vi "MenuSelection(User).vi"(6 "User events":T8, 8 "error in":errorcluster {"code" min=0 max=0}, 10 "ItemTag":string, 11 "Data in":T1={"Class"={"Ants"=refnum, "Layer"=refnum, "Templates"=refnum, "Icon"=refnum, "Glyph"=refnum, "Settings"=refnum, "Tools"=refnum}, "Ref"={"Add Layer"=refnum, "Remove Layer"=refnum, "Line Text"=[], "Body Text Spec"=refnum, "DNL_Font"=refnum, "glyph path str"=refnum, "templates path str"=refnum, "Arrow Up"=refnum, "Arrow Down"=refnum, "IE VI Ref"=refnum, "Glyphs tree"=refnum, "Templates tree"=refnum, "Layer Icon Text"=refnum, "Layer Template"=refnum, "Clipboard"=refnum, "BW icon in"=refnum, "Color icon in"=refnum, "Layer Clust"=refnum, "Body Text"=refnum, "DNL_Framework Templates"=refnum, "Search Templates"=refnum, "TextMarker"=refnum, "Tab Control"=refnum, "Search Glyphs"=refnum, "Line Color"=refnum, "DNL_Glyphs []"=refnum, "Fill Color"=refnum, "Tools"=refnum, "Glyphs tree"=refnum, "Icon"=refnum, "Preview"=refnum, "Ants"=refnum, "Terminals"=refnum, "menu reference"=refnum, "LayerNames"=[], "GlyphLoadAnimation"=refnum, "TemplateLoadAnimation"=refnum, "refreshGlyphs"=refnum, "refreshTemplates"=refnum}, "Support"={"AntsRect"={"left"=0, "top"=0, "right"=0, "bottom"=0}, "Mouse Move Coords"={"Horizontal"=0, "Vertical"=0}, "Mouse Down Coords"={"Horizontal"=0, "Vertical"=0}, "Temp Coord"={"Horizontal"=0, "Vertical"=0}, "Action"=enum."Default", "Edge Color"=4914962, "Fill Color"=16860, "Mouse Down?"=FALSE, "Draft Mode?"=FALSE, "Temp Icon"=bytes[3102], "CTRL Pressed"=FALSE, "Move Selection?"=FALSE, "AntsRect Orig"={"left"=0, "top"=0, "right"=0, "bottom"=0}, "Text"="", "TM Set?"=FALSE, "Mouse inside icon?"=FALSE, "Tool (old value)"=0, "Pencil Move Color"=0, "Swap Colors?"=FALSE, "Shift pressed?"=FALSE}}) -> (0 "error out":errorcluster {"code" min=0 max=0}, 3 "Data out":T1={"Class"={"Ants"=refnum, "Layer"=refnum, "Templates"=refnum, "Icon"=refnum, "Glyph"=refnum, "Settings"=refnum, "Tools"=refnum}, "Ref"={"Add Layer"=refnum, "Remove Layer"=refnum, "Line Text"=[], "Body Text Spec"=refnum, "DNL_Font"=refnum, "glyph path str"=refnum, "templates path str"=refnum, "Arrow Up"=refnum, "Arrow Down"=refnum, "IE VI Ref"=refnum, "Glyphs tree"=refnum, "Templates tree"=refnum, "Layer Icon Text"=refnum, "Layer Template"=refnum, "Clipboard"=refnum, "BW icon in"=refnum, "Color icon in"=refnum, "Layer Clust"=refnum, "Body Text"=refnum, "DNL_Framework Templates"=refnum, "Search Templates"=refnum, "TextMarker"=refnum, "Tab Control"=refnum, "Search Glyphs"=refnum, "Line Color"=refnum, "DNL_Glyphs []"=refnum, "Fill Color"=refnum, "Tools"=refnum, "Glyphs tree"=refnum, "Icon"=refnum, "Preview"=refnum, "Ants"=refnum, "Terminals"=refnum, "menu reference"=refnum, "LayerNames"=[], "GlyphLoadAnimation"=refnum, "TemplateLoadAnimation"=refnum, "refreshGlyphs"=refnum, "refreshTemplates"=refnum}, "Support"={"AntsRect"={"left"=0, "top"=0, "right"=0, "bottom"=0}, "Mouse Move Coords"={"Horizontal"=0, "Vertical"=0}, "Mouse Down Coords"={"Horizontal"=0, "Vertical"=0}, "Temp Coord"={"Horizontal"=0, "Vertical"=0}, "Action"=enum."Default", "Edge Color"=4914962, "Fill Color"=16860, "Mouse Down?"=FALSE, "Draft Mode?"=FALSE, "Temp Icon"=bytes[3102], "CTRL Pressed"=FALSE, "Move Selection?"=FALSE, "AntsRect Orig"={"left"=0, "top"=0, "right"=0, "bottom"=0}, "Text"="", "TM Set?"=FALSE, "Mouse inside icon?"=FALSE, "Tool (old value)"=0, "Pencil Move Color"=0, "Swap Colors?"=FALSE, "Shift pressed?"=FALSE}})   [LabVIEW 2021]
uses:
  Controls/IE Data.ctl
  Class/Ants/Ants.lvclass
  Class/FakedArray/FakedArray.lvclass
  vi.lib/LabVIEW Icon API/lv_icon/Classes/Icon/Icon.lvclass
  Class/Icon Library/Glyph.lvclass
  Class/Settings/Settings.lvclass
  Class/Tools/Tools Paint.lvclass
  Controls/IE Classes.ctl
  Controls/References Cluster.ctl
  Controls/SupportClass.ctl
  <vilib>/Utility/miscctls.llb/LVPoint32TypeDef.ctl
  Controls/SupportClass_Action.ctl
  vi.lib/LabVIEW Icon API/lv_icon/Controls/IEColor.ctl
  vi.lib/LabVIEW Icon API/lv_icon/Controls/Pathes.ctl
  vi.lib/LabVIEW Icon API/lv_icon/Controls/Graphic.ctl
  vi.lib/LabVIEW Icon API/lv_icon/Classes/Icon Framework/Icon Framework.lvclass
  vi.lib/LabVIEW Icon API/lv_icon/Classes/Layer/Layer.lvclass
  vi.lib/LabVIEW Icon API/lv_icon/Controls/Layer.ctl
  Controls/Undo Redo Action.ctl
  Controls/Tools.ctl
  vi.lib/LabVIEW Icon API/lv_icon/lv_icon.lvlib
panel:
  in  "Layer name":string="Clipboard"
  in  "glyph":string="Glyph name"
  in  "template":string="Template name"
  in  "Prompt":string="Save Glyph"
  in  "prompt":string="Save Icon Template"
  in  "LayerName":string="Merged Layers"
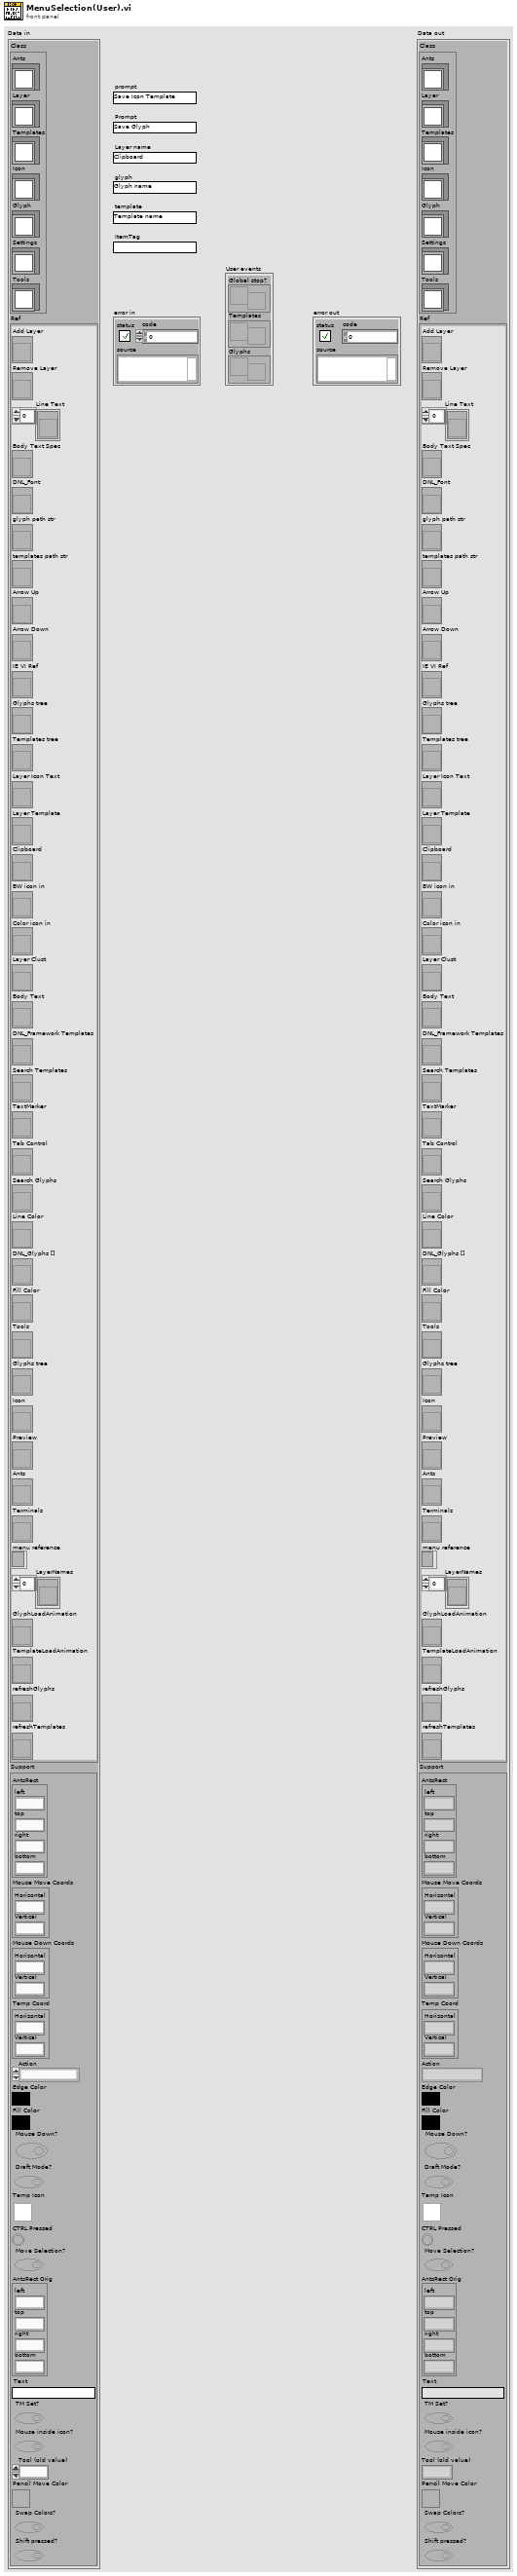
[diagram p1: front panel]
types:
  T1 = typedef "IE Data.ctl" = cluster{"Class":T2, "Ref":T3, "Support":T4}
  T2 = typedef "IE Classes.ctl" = cluster{"Ants":refnum<class "Ants.lvclass">, "Layer":refnum<class "FakedArray.lvclass">, "Templates":refnum<class "FakedArray.lvclass">, "Icon":refnum<class "Icon.lvclass">, "Glyph":refnum<class "Glyph.lvclass">, "Settings":refnum<class "Settings.lvclass">, "Tools":refnum<class "Tools Paint.lvclass">}
  T3 = typedef "References Cluster.ctl" = cluster{"Add Layer":refnum<vi>, "Remove Layer":refnum<vi>, "Line Text":refnum<vi>[], "Body Text Spec":refnum<vi>, "DNL_Font":refnum<vi>, "glyph path str":refnum<vi>, "templates path str":refnum<vi>, "Arrow Up":refnum<vi>, "Arrow Down":refnum<vi>, "IE VI Ref":refnum<vi>, "Glyphs tree":refnum<vi>, "Templates tree":refnum<vi>, "Layer Icon Text":refnum<vi>, "Layer Template":refnum<vi>, "Clipboard":refnum<vi>, "BW icon in":refnum<vi>, "Color icon in":refnum<vi>, "Layer Clust":refnum<vi>, "Body Text":refnum<vi>, "DNL_Framework Templates":refnum<vi>, "Search Templates":refnum<vi>, "TextMarker":refnum<vi>, "Tab Control":refnum<vi>, "Search Glyphs":refnum<vi>, "Line Color":refnum<vi>, "DNL_Glyphs []":refnum<vi>, "Fill Color":refnum<vi>, "Tools":refnum<vi>, "Glyphs tree":refnum<vi>, "Icon":refnum<vi>, "Preview":refnum<vi>, "Ants":refnum<vi>, "Terminals":refnum<vi>, "menu reference":refnum<k9>, "LayerNames":refnum<vi>[], "GlyphLoadAnimation":refnum<vi>, "TemplateLoadAnimation":refnum<vi>, "refreshGlyphs":refnum<vi>, "refreshTemplates":refnum<vi>}
  T4 = typedef "SupportClass.ctl" = cluster{"AntsRect":cluster{"left":i16, "top":i16, "right":i16, "bottom":i16}, "Mouse Move Coords":T5, "Mouse Down Coords":T5, "Temp Coord":T5, "Action":T6, "Edge Color":T7, "Fill Color":T7, "Mouse Down?":bool, "Draft Mode?":bool, "Temp Icon":picture, "CTRL Pressed":bool, "Move Selection?":bool, "AntsRect Orig":cluster{"left":i16, "top":i16, "right":i16, "bottom":i16}, "Text":string, "TM Set?":bool, "Mouse inside icon?":bool, "Tool (old value)":u32, "Pencil Move Color":u32, "Swap Colors?":bool, "Shift pressed?":bool}
  T5 = typedef "LVPoint32TypeDef.ctl" = cluster{"Horizontal":i32, "Vertical":i32}
  T6 = typedef "SupportClass_Action.ctl" = enum16{"Default", "Move Selection", "Glyph Library", "Tool"}
  T7 = typedef "IEColor.ctl" = u32
  T8 = cluster{"Global stop?":refnum<user-event>, "Templates":refnum<user-event>, "Glyphs":refnum<user-event>}
  T9 = typedef "Pathes.ctl" = enum16{"Root Path", "Icon Templates", "Icon Templates VI", "Icon Templates Lib", "Glyphs"}
  T10 = typedef "Graphic.ctl" = cluster{"Rectangle":cluster{"left":i16, "top":i16, "right":i16, "bottom":i16}, "Path":path, "Image":picture, "Filter":string, "FileName":string}
  T11 = typedef "Layer.ctl" = cluster{"LayerIcon":picture, "LayerName":string, "Opacity":u8, "Visibility?":bool}
  T12 = typedef "Undo Redo Action.ctl" = enum16{"Init", "Add", "Redo", "Undo", "Undo Preview"}
  T13 = enum32{"Pencil", "Line", "Dropper", "Fill", "Rectangle", "Filled Rectangle", "Ellipse", "Filled Ellipse", "Eraser", "Text", "Select", "Move"}
  T14 = typedef "Tools.ctl" = enum32{"Pencil", "Line", "Dropper", "Fill", "Rectangle", "Filled Rectangle", "Ellipse", "Filled Ellipse", "Eraser", "Text", "Select", "Move"}
  T15 = typedef "imagedata.ctl" = cluster{"image type":i32, "image depth":i32, "image":u8[], "mask":u8[], "colors":u32[], "Rectangle":cluster{"left":i16, "top":i16, "right":i16, "bottom":i16}}
  T16 = typedef "Font.ctl" = string
  T17 = typedef "Alignment.ctl" = u16
  T18 = typedef "Font Size.ctl" = u8
  T19 = cluster{"Line 1 text":string, "Line 2 text":string, "Line 3 text":string, "Line 4 text":string, "Line 1 color":u32, "Line 2 color":u32, "Line 3 color":u32, "Line 4 color":u32, "Body Text Spec":cluster{"DNL_Font":T16, "Alignment":T17, "Size":T18}, "Center text vertically":bool, "Capitalize Text":bool}
  T20 = cluster{"left":i16, "top":i16, "right":i16, "bottom":i16}
  T21 = cluster{"Horizontal":i32, "Vertical":i32, "Vertical 2":i32, "Vertical 3":i32}
  T22 = cluster{"Left":i32, "Top":i32, "Right":i32, "Bottom":i32}
  T23 = typedef "Icon Editor Invoker Type.ctl" = enum32{"Unknown Icon Source", "VI Icon", "Library Icon (any library type)", "Palette icon", "Icon from App Method"}
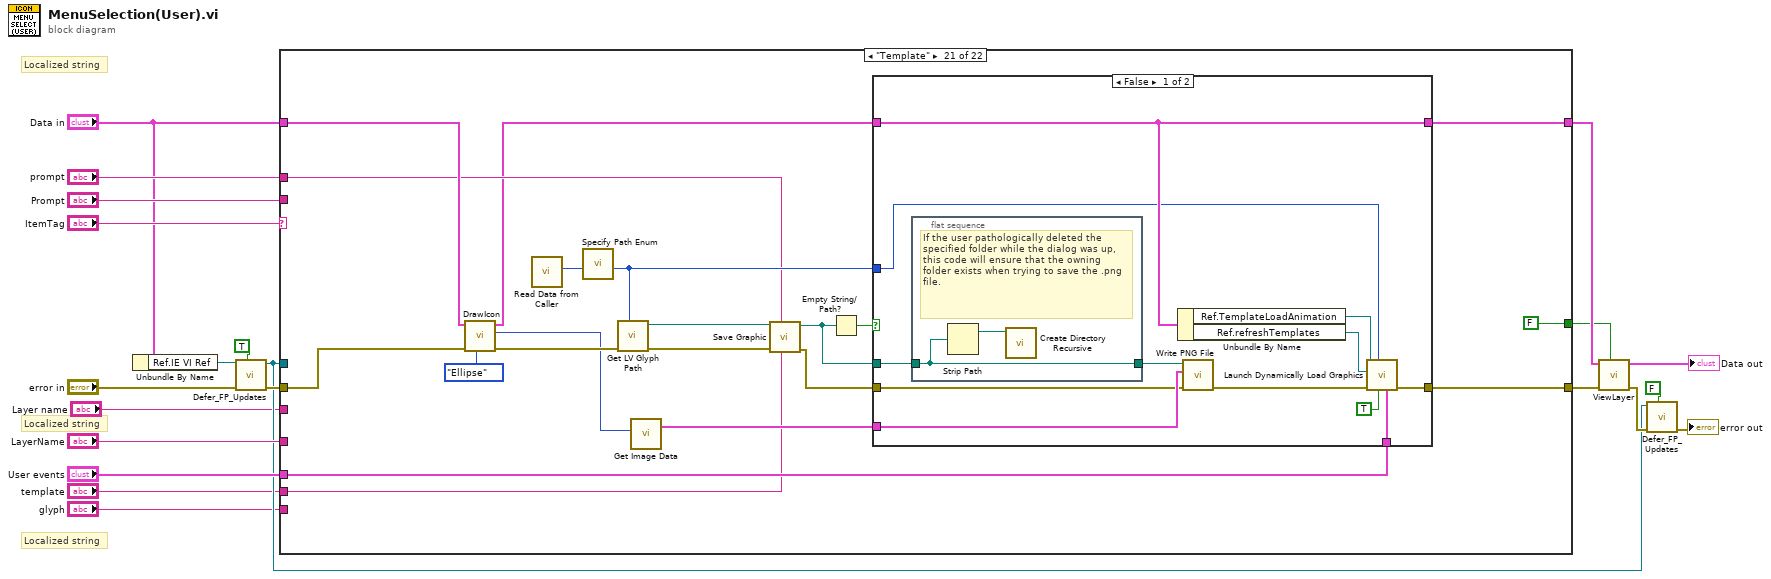
[diagram p0: block diagram]
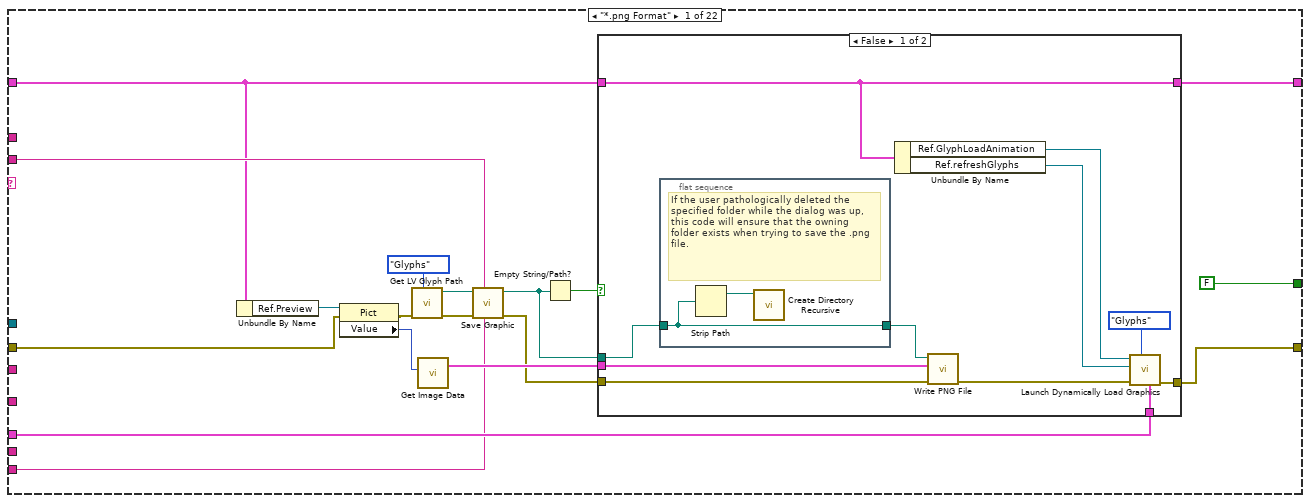
[diagram p2: hidden frame]
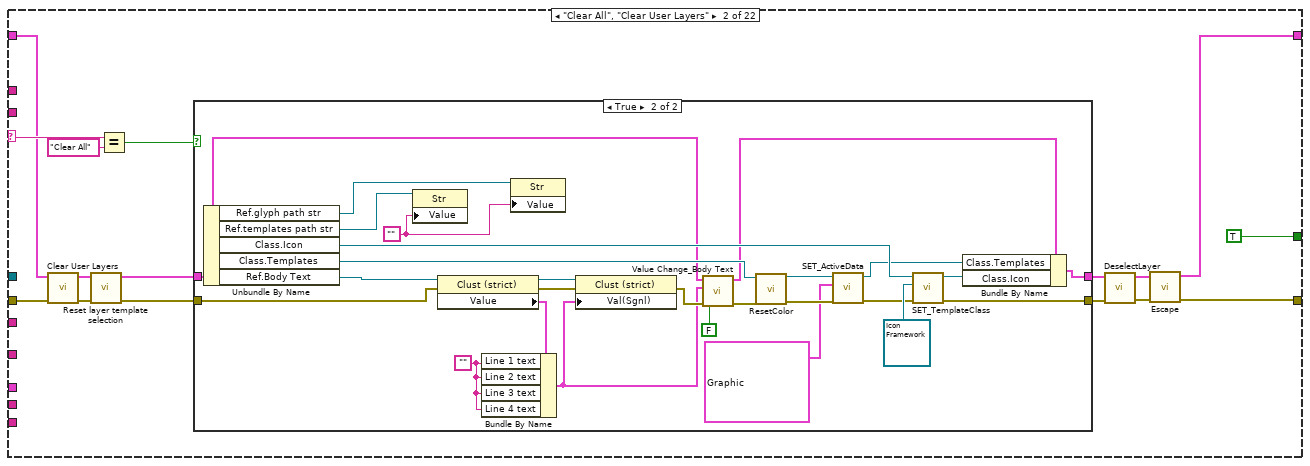
[diagram p4: hidden frame]
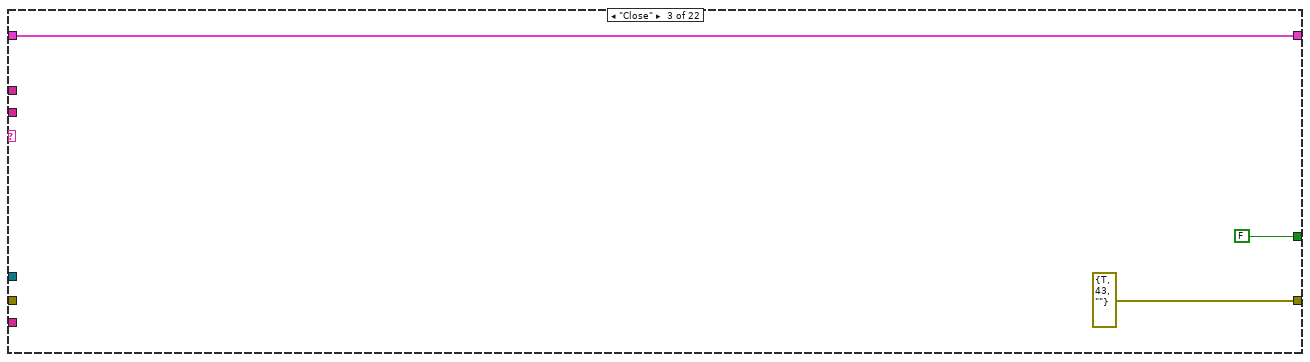
[diagram p6: hidden frame]
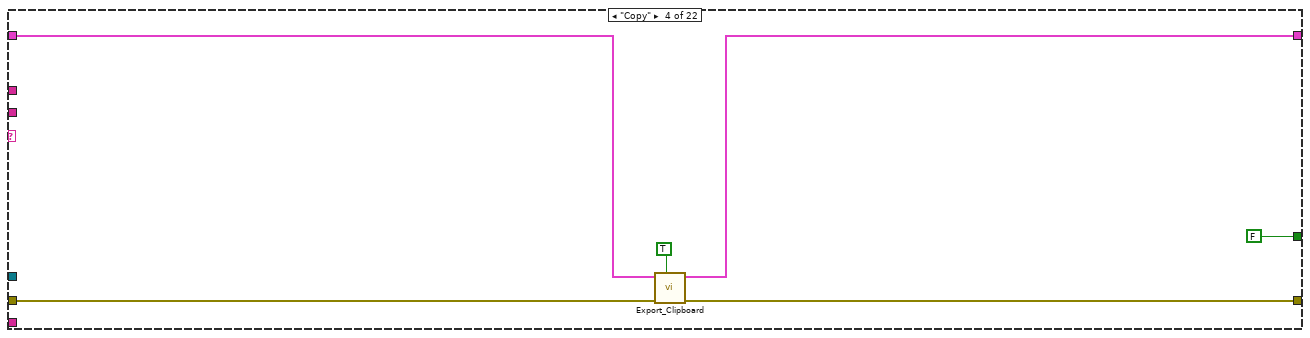
[diagram p7: hidden frame]
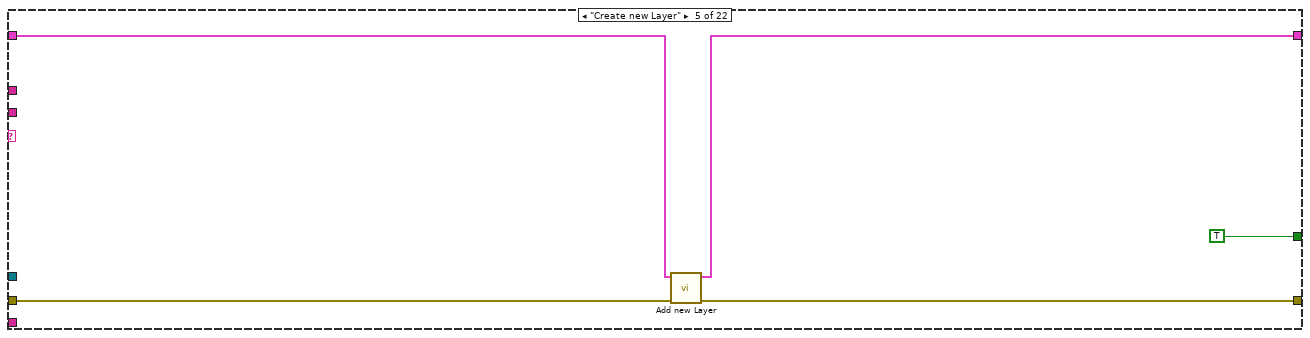
[diagram p8: hidden frame]
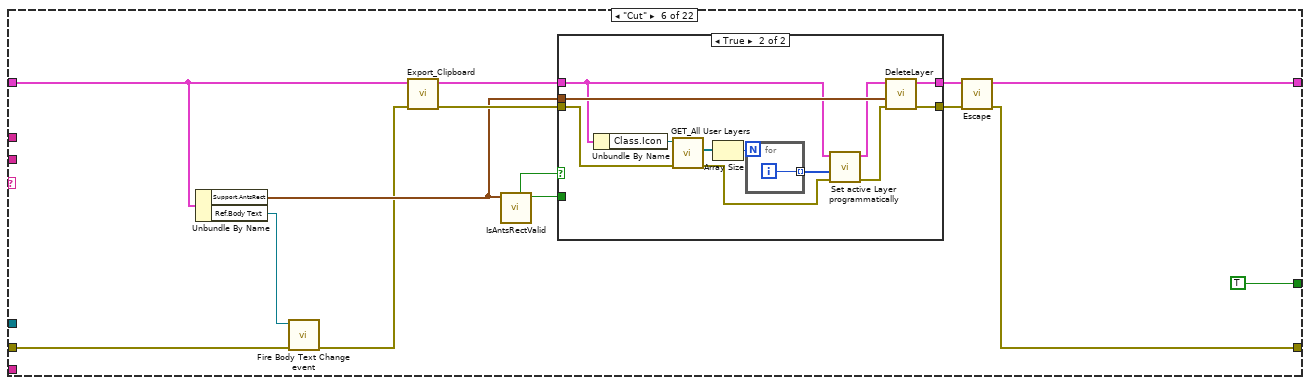
[diagram p9: hidden frame]
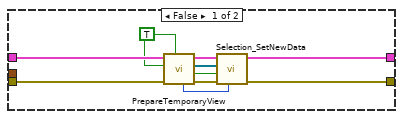
[diagram p10: hidden frame]
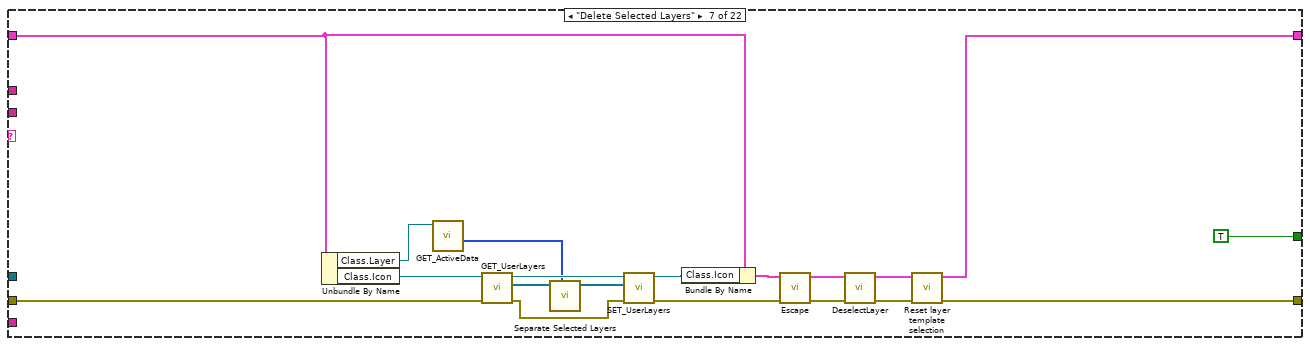
[diagram p11: hidden frame]
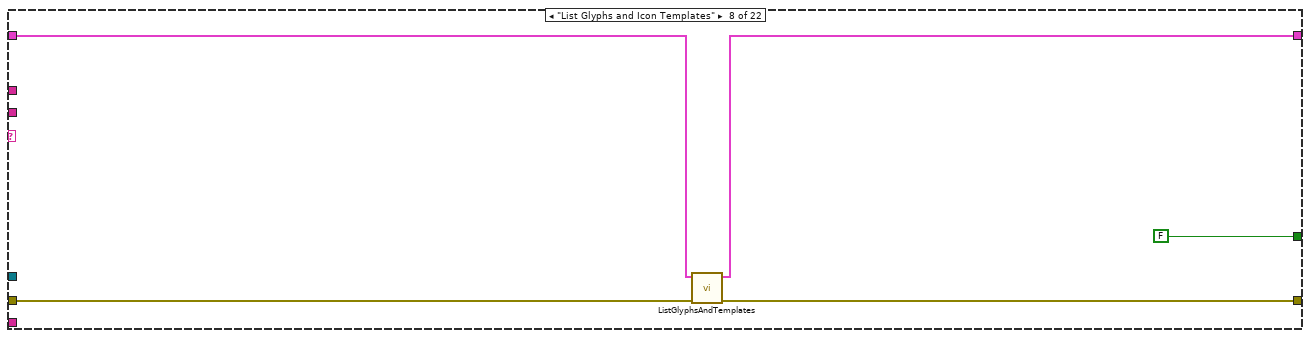
[diagram p12: hidden frame]
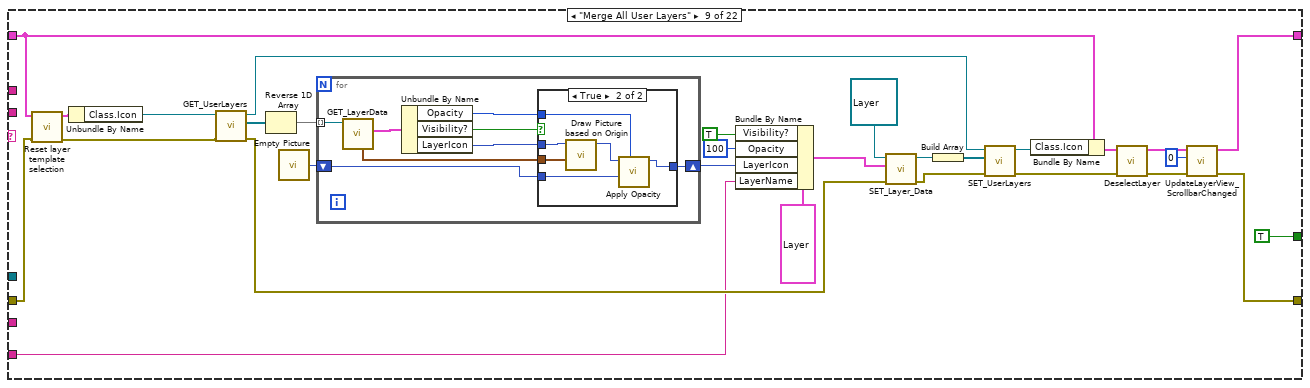
[diagram p13: hidden frame]
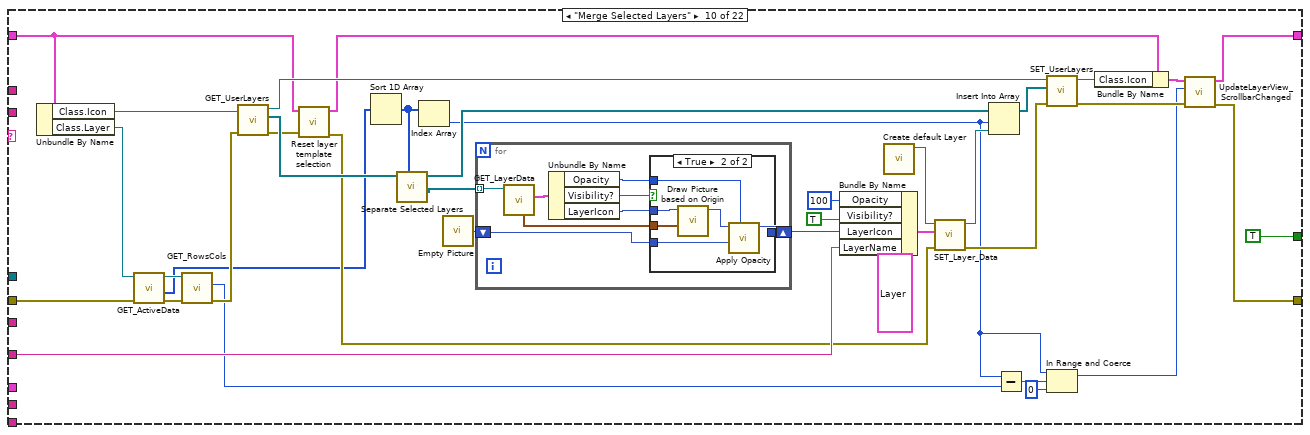
[diagram p15: hidden frame]
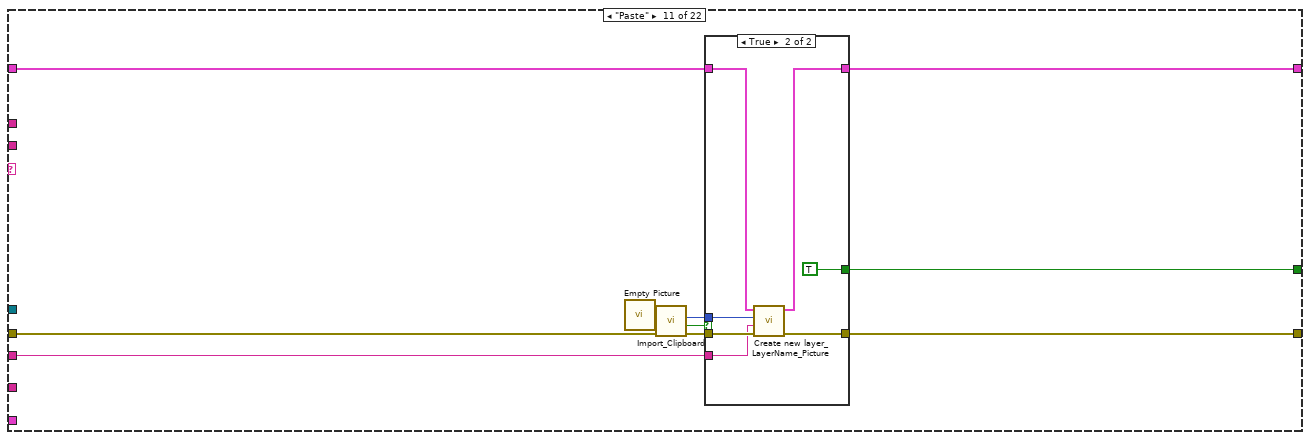
[diagram p17: hidden frame]
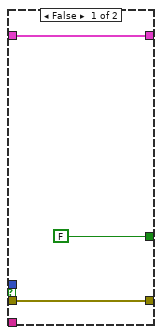
[diagram p18: hidden frame]
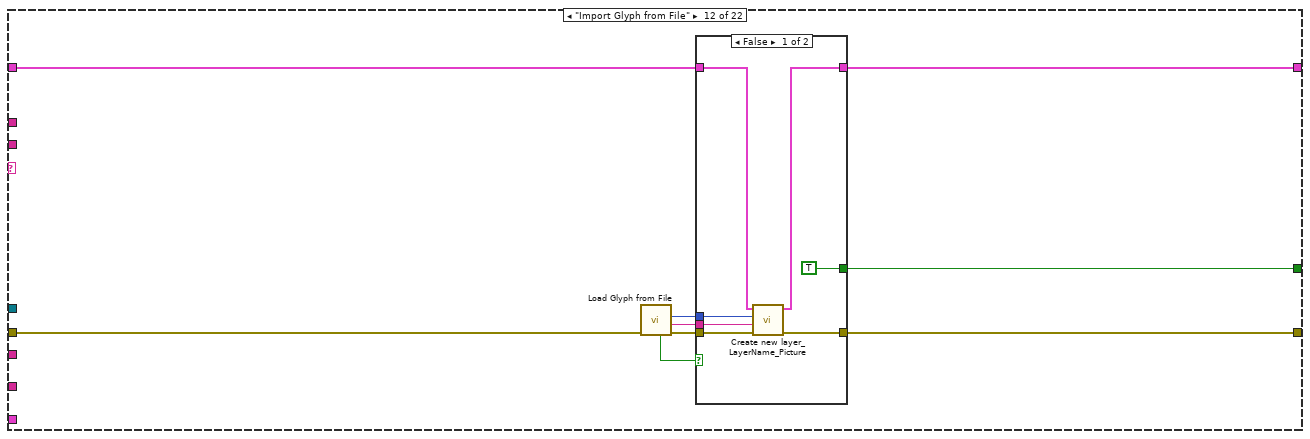
[diagram p19: hidden frame]
diagram:
  # "Localized string"
  # "Localized string"
  # "Localized string"
  n1 = Unbundle By Name("Data in") -> ("Ref.IE VI Ref"=w8:refnum<vi>)
  n2 = call "Defer_FP_Updates.vi"("Defer Panel Updates"=TRUE, "error in (no error)"="error in", "lv_icon.vi in"=w8) -> ("error out"=w11:errorcluster, "lv icon.vi out"=w4:refnum<vi>)  [unwired: 7 out]
  n3 = case shown="\"Template\"" "ItemTag" {
    selector: "ItemTag" -> [_ w70 _ _ _ _ _ _ _ _ _ _ _ w340 _ w388 _ _ _ _ _ _]
    tunnel: w11 -> [w26 w59 _ w107 w108 w115 w160 w173 w188 w219 w275 w296 w321 w325 w373 w378 w397 w400 w415 w438 w461 w493]
    tunnel: [w27 w62 errorcluster {"status"=TRUE, "code"=43, "source"=""} ("Icon 43") w106 w109 w125 w150 w172 w175 w231 w278 w298 w312 w331 w354 w380 w390 w402 w416 w445 w460 w493] -> w16
    tunnel: "LayerName" -> [_ _ _ _ _ _ _ _ w190 w244 _ _ _ _ _ _ _ _ _ _ _ _]
    tunnel: "prompt" -> [_ _ _ _ _ _ _ _ _ _ _ _ _ _ _ _ _ _ _ _ w463 _]
    tunnel: "Prompt" -> [w28 _ _ _ _ _ _ _ _ _ _ _ _ _ _ _ _ _ _ _ _ _]
    tunnel: [FALSE TRUE FALSE FALSE TRUE TRUE TRUE FALSE TRUE TRUE w280 w291 TRUE FALSE FALSE FALSE FALSE FALSE FALSE FALSE FALSE FALSE] -> w13
    tunnel: "User events" -> [w33 _ _ _ _ _ _ _ _ _ _ _ _ _ _ _ _ _ _ w443 w469 _]
    tunnel: [w22 w63 w99 w104 w111 w124 w153 w169 w176 w233 w277 w297 w309 w323 w355 w379 w389 w403 w414 w429 w456 w491] -> w14
    tunnel: "Data in" -> [w23 w60 w99 w103 w110 w119 w155 w170 w184 w236 w279 w299 w311 w327 w369 w381 w396 w405 w419 w430 w466 w491]
    tunnel: w4 -> [_ _ _ _ _ _ _ _ _ _ _ _ _ _ _ _ _ w399 _ _ _ _]
    tunnel: "template" -> [_ _ _ _ _ _ _ _ _ _ _ _ _ _ _ _ _ _ _ _ w458 _]
    tunnel: "glyph" -> [w24 _ _ _ _ _ _ _ _ _ _ _ _ _ _ _ _ _ _ _ _ _]
    tunnel: "Layer name" -> [_ _ _ _ _ _ _ _ _ _ w271 _ _ _ _ _ _ _ _ _ _ _]
    frame "*.png Format" {
      n4 = Unbundle By Name(w23) -> ("Ref.Preview"=w39:refnum<vi>)
      n5 = property class="Pict"(reference=w39, error in=w26) -> (error out=w35:errorcluster, "Value"=w37:picture)  [unwired: 1 out]
      n6 = call "Get LV Glyph Path.vi"("Path"=Pathes."Glyphs", "error in (no error)"=w35) -> ("error out"=w32:errorcluster, "Requested Path"=w29:path)  [unwired: 1 in, 7 out]
      n7 = call "Get Image Data.vi"("Pic In"=w37) -> ("image data out"=w38:T15)  [unwired: 3 in, 7 out]
      n8 = call "Save Graphic.vi"("Loc string caption"=w24, "FP Title"=w28, "error in (no error)"=w32, "Start path in"=w29) -> ("error out"=w31:errorcluster, "Output"=w30:path)  [unwired: 6 out]
      n9 = Empty String/Path?(string/path=w30) -> (empty?=w25:bool)
      n10 = case shown="False" w25 {
        tunnel: w38 -> [w50 _]
        tunnel: w33 -> [w47 _]
        tunnel: w31 -> [w46 w54]
        tunnel: w30 -> [w41 _]
        tunnel: [w45 w54] -> w27
        tunnel: w23 -> [w44 w53]
        tunnel: [w44 w53] -> w22
        frame False {
          n11 = flat-sequence {
            tunnel: w41 -> [w52]
            tunnel: [w52] -> w40
            frame #0 {
              # "If the user pathologically deleted the specified folder while the dialog was up, this code will ensure that the owning folder exists when trying to save the .png file."
              n12 = Strip Path(path=w52) -> (stripped path=w51:path)  [unwired: 1 out]
              n13 = call <vilib>:"Create Directory Recursive.vi"("directory"=w51) -> ()  [unwired: 4 in, 3 out]
            }
          }
          n14 = Unbundle By Name(w44) -> ("Ref.GlyphLoadAnimation"=w42:refnum<vi>, "Ref.refreshGlyphs"=w43:refnum<vi>)
          n15 = call <vilib>:"Write PNG File.vi"("error in (no error)"=w46, "image data"=w50, "path to PNG file"=w40) -> ("error out"=w49:errorcluster)  [unwired: 1 in, 7 out]
          n16 = call "Launch Dynamically Load Graphics.vi"("User events"=w47, "Path"=Pathes."Glyphs", "error in (no error)"=w49, "button ref"=w43, "animatedDecoration ref"=w42) -> ("error out"=w45:errorcluster)  [unwired: 1 in, 5 out]
        }
        frame True {
        }
      }
    }
    frame "Clear All", "Clear User Layers" {
      n17 = call "Clear User Layers.vi"("error in"=w59, "Data in"=w60) -> ("error out"=w58:errorcluster, "Data out"=w57:T1)  [unwired: 8 out]
      n18 = call "Reset layer template selection.vi"("error in (no error)"=w58, "Data in"=w57) -> ("error out"=w55:errorcluster, "Data out"=w56:T1)  [unwired: 1 in, 7 out]
      n19 = Equal?(x=w70, y="Clear All") -> (x = y?=w69:bool)
      n20 = case shown="True" w69 {
        tunnel: w55 -> [w72 w86]
        tunnel: w56 -> [w71 w77]
        tunnel: [w72 w80] -> w67
        tunnel: [w71 w78] -> w65
        frame False {
        }
        frame True {
          w73 = ""
          w94 = ""
          n21 = Unbundle By Name(w77) -> ("Ref.glyph path str"=w74:refnum<vi>, "Ref.templates path str"=w75:refnum<vi>, "Class.Icon"=w83:refnum<class "Icon.lvclass">, "Class.Templates"=w85:refnum<class "FakedArray.lvclass">, "Ref.Body Text"=w98:refnum<vi>)
          n22 = property class="Str"(reference=w75, "Value"=w73) -> ()  [unwired: 1 in, 2 out]
          n23 = property class="Clust (strict)"(reference=w98, error in=w86) -> (reference out=w97:refnum<vi>, error out=w96:errorcluster, "Value"=w95:T19)
          n24 = Bundle By Name(cluster=w95, "Line 1 text"=w94, "Line 2 text"=w94, "Line 3 text"=w94, "Line 4 text"=w94) -> (w87:T19)
          n25 = property class="Str"(reference=w74, "Value"=w73) -> ()  [unwired: 1 in, 2 out]
          n26 = property class="Clust (strict)"(reference=w97, error in=w96, "Val(Sgnl)"=w87) -> (error out=w89:errorcluster)  [unwired: 1 out]
          n27 = call "Value Change_Body Text.vi"("Add to Undo?"=FALSE, "error in"=w89, "NewVal"=w87, "Data in"=w77) -> ("error out"=w84:errorcluster, "Data out"=w76:T1)  [unwired: 1 in, 5 out]
          n28 = call "ResetColor.vi"("error in (no error)"=w84, "FakedArray in"=w85) -> ("error out"=w92:errorcluster, "FakedArray out"=w93:refnum<class "FakedArray.lvclass">)  [unwired: 8 out]
          n29 = call-dynamic "SET_ActiveData.vi"("error in (no error)"=w92, "Active Data"=T10 {"Rectangle"={"left"=0, "top"=0, "right"=0, "bottom"=0}, "Path"=path "", "Image"=bytes[0], "Filter"="", "FileName"=""} ("Path & Icon"), "FakedArray.lvclass in"=w93) -> ("error out"=w82:errorcluster, "FakedArray.lvclass out"=w79:refnum<class "FakedArray.lvclass">)  [unwired: 7 out]
          n30 = call-dynamic "SET_TemplateClass.vi"("error in (no error)"=w82, "Icon Framework.lvclass"=refnum<class "Icon Framework.lvclass"> refnum ("lv_icon.lvlib:Icon Framework.lvclass"), "Icon.lvclass in"=w83) -> ("error out"=w80:errorcluster, "Icon.lvclass out"=w81:refnum<class "Icon.lvclass">)  [unwired: 7 out]
          n31 = Bundle By Name(cluster=w76, "Class.Templates"=w79, "Class.Icon"=w81) -> (w78:T1)
        }
      }
      n32 = call "DeselectLayer.vi"("error in (no error)"=w67, "Data in"=w65) -> ("error out"=w61:errorcluster, "Data out"=w64:T1)  [unwired: 8 out]
      n33 = call "Escape.vi"("error in"=w61, "Data in"=w64) -> ("error out"=w62:errorcluster, "Data out"=w63:T1)  [unwired: 2 in, 6 out]
    }
    frame "Close" {
    }
    frame "Copy" {
      n34 = call "Export_Clipboard.vi"("Is Copy? (F)"=TRUE, "error in (no error)"=w107, "Data in"=w103) -> ("error out"=w106:errorcluster, "Data out"=w104:T1)  [unwired: 7 out]
    }
    frame "Create new Layer" {
      n35 = call "Add new Layer.vi"("error in"=w108, "Data in"=w110) -> ("error out"=w109:errorcluster, "Data out"=w111:T1)  [unwired: 8 out]
    }
    frame "Cut" {
      n36 = Unbundle By Name(w119) -> ("Support.AntsRect"=w118:T20, "Ref.Body Text"=w116:refnum<vi>)
      n37 = call "Fire Body Text Change event.vi"("error in"=w115, "Ref.Body Text"=w116) -> ("error out"=w114:errorcluster)  [unwired: 2 in, 7 out]
      n38 = call "Export_Clipboard.vi"("error in (no error)"=w114, "Data in"=w119) -> ("error out"=w121:errorcluster, "Data out"=w120:T1)  [unwired: 8 out]
      n39 = call "IsAntsRectValid.vi"("AntsRect"=w118) -> ("Valid?"=w122:bool, "Max. Rect size?"=w123:bool)  [unwired: 9 out]
      n40 = case shown="True" w123 {
        tunnel: w122 -> [_ _]
        tunnel: w120 -> [w136 w140]
        tunnel: [w135 w147] -> w113
        tunnel: [w134 w148] -> w117
        tunnel: w121 -> [w127 w138]
        tunnel: w118 -> [_ w146]
        frame False {
          w133 = TRUE ("Delete Selected Area?")
          n41 = call "PrepareTemporaryView.vi"("Delete Selected Area?"=w133, "error in (no error)"=w127, "Valid Selection?"=w133, "Data in"=w136) -> ("error out"=w130:errorcluster, "Highlighted?"=w131:bool, "All Layers out"=w132:refnum<class "Layer.lvclass">[], "Data out"=w128:T1, "#Active Layer"=w129:i32)  [unwired: 1 in, 2 out]
          n42 = call "Selection_SetNewData.vi"("#Active Layer"=w129, "error in"=w130, "Highlighted?"=w131, "All Layers In"=w132, "Data in"=w128) -> ("error out"=w135:errorcluster, "Data out"=w134:T1)  [unwired: 1 in, 3 out]
        }
        frame True {
          n43 = Unbundle By Name(w140) -> ("Class.Icon"=w145:refnum<class "Icon.lvclass">)
          n44 = call-dynamic "GET_All User Layers.vi"("error in (no error)"=w138, "Icon.lvclass in"=w145) -> ("error out"=w144:errorcluster, "User Layer"=w141:refnum<class "Layer.lvclass">[])  [unwired: 7 in, 1 out]
          n45 = Array Size(array=w141) -> (size(s)=w142:i32)
          n46 = for {
            N: w142 -> [_]
            tunnel: [w149] -> w143 mode=indexing
            i -> [w149]
          }
          n47 = call "Set active Layer programmatically.vi"("error in"=w144, "Active Layer []"=w143, "Data in"=w140) -> ("error out"=w137:errorcluster, "Data out"=w139:T1)  [unwired: 7 in]
          n48 = call "DeleteLayer.vi"("error in"=w137, "AntsRect"=w146, "Data in"=w139) -> ("error out"=w147:errorcluster, "Data out"=w148:T1)  [unwired: 5 out]
        }
      }
      n49 = call "Escape.vi"("error in"=w113, "Data in"=w117) -> ("error out"=w125:errorcluster, "Data out"=w124:T1)  [unwired: 2 in, 6 out]
    }
    frame "Delete Selected Layers" {
      n50 = Unbundle By Name(w155) -> ("Class.Layer"=w152:refnum<class "FakedArray.lvclass">, "Class.Icon"=w163:refnum<class "Icon.lvclass">)
      n51 = call-dynamic "GET_ActiveData.vi"("FakedArray in"=w152) -> ("Active Data []"=w161:i32[])  [unwired: 1 in, 9 out]
      n52 = call-dynamic "GET_UserLayers.vi"("error in (no error)"=w160, "Icon.lvclass in"=w163) -> ("error out"=w164:errorcluster, "All Layers"=w168:refnum<class "Layer.lvclass">[], "Icon.lvclass out"=w167:refnum<class "Icon.lvclass">)  [unwired: 7 out]
      n53 = call "Separate Selected Layers.vi"("Active Indices"=w161, "All Layers"=w168) -> ("Layers out not in Array"=w166:refnum<class "Layer.lvclass">[])  [unwired: 9 out]
      n54 = call-dynamic "SET_UserLayers.vi"("error in (no error)"=w164, "Layers"=w166, "Icon.lvclass in"=w167) -> ("error out"=w151:errorcluster, "Icon.lvclass out"=w162:refnum<class "Icon.lvclass">)  [unwired: 7 in]
      n55 = Bundle By Name(cluster=w155, "Class.Icon"=w162) -> (w154:T1)
      n56 = call "Escape.vi"("error in"=w151, "Data in"=w154) -> ("error out"=w159:errorcluster, "Data out"=w158:T1)  [unwired: 8 out]
      n57 = call "DeselectLayer.vi"("error in (no error)"=w159, "Data in"=w158) -> ("error out"=w156:errorcluster, "Data out"=w157:T1)  [unwired: 8 out]
      n58 = call "Reset layer template selection.vi"("error in (no error)"=w156, "Data in"=w157) -> ("error out"=w150:errorcluster, "Data out"=w153:T1)  [unwired: 1 in, 7 out]
    }
    frame "List Glyphs and Icon Templates" {
      n59 = call "ListGlyphsAndTemplates.vi"("error in"=w173, "Data in"=w170) -> ("error out"=w172:errorcluster, "Data out"=w169:T1)  [unwired: 8 out]
    }
    frame "Merge All User Layers" {
      n60 = call "Reset layer template selection.vi"("error in (no error)"=w188, "Data in"=w184) -> ("error out"=w187:errorcluster, "Data out"=w186:T1)  [unwired: 1 in, 7 out]
      n61 = Unbundle By Name(w186) -> ("Class.Icon"=w185:refnum<class "Icon.lvclass">)
      n62 = call-dynamic "GET_UserLayers.vi"("error in (no error)"=w187, "Icon.lvclass in"=w185) -> ("error out"=w194:errorcluster, "All Layers"=w202:refnum<class "Layer.lvclass">[], "Icon.lvclass out"=w201:refnum<class "Icon.lvclass">)  [unwired: 7 out]
      n63 = Reverse 1D Array(array=w202) -> (reversed array=w192:refnum<class "Layer.lvclass">[])
      n64 = call "Empty Picture"() -> ("empty picture"=w191:picture)
      n65 = for {
        shift-right: [w207] -> w198
        shift-left: w191 -> [w208]
        tunnel: w192 -> [w203] mode=indexing
        n66 = call-dynamic "GET_LayerData.vi"("Layer.lvclass in"=w203) -> ("Data"=w205:T11, "Origin"=w204:T5)  [unwired: 1 in, 8 out]
        n67 = Unbundle By Name(w205) -> ("Opacity"=w209:u8, "Visibility?"=w210:bool, "LayerIcon"=w206:picture)
        n68 = case shown="True" w210 {
          tunnel: w209 -> [_ w217]
          tunnel: w208 -> [w211 w216]
          tunnel: [w211 w215] -> w207
          tunnel: w206 -> [_ w214]
          tunnel: w204 -> [_ w213]
          frame False {
          }
          frame True {
            n69 = call "Draw Picture based on Origin.vi"("Origin"=w213, "LayerIcon in"=w214) -> ("LayerIcon out"=w212:picture)  [unwired: 1 in, 8 out]
            n70 = call "Apply Opacity.vi"("% (100)"=w217, "Bottom"=w216, "Top"=w212) -> ("new picture"=w215:picture)  [unwired: 8 out]
          }
        }
      }
      n71 = Bundle By Name(cluster=T11 {"LayerIcon"=bytes[0], "LayerName"="", "Opacity"=0, "Visibility?"=FALSE} ("Data"), "Visibility?"=TRUE, "Opacity"=u8 100, "LayerIcon"=w198, "LayerName"=w190) -> (w197:T11)
      n72 = call-dynamic "SET_Layer_Data.vi"("error in (no error)"=w194, "Data"=w197, "Layer.lvclass in"=refnum<class "Layer.lvclass"> refnum) -> ("error out"=w195:errorcluster, "Layer.lvclass out"=w200:refnum<class "Layer.lvclass">)  [unwired: 1 in, 6 out]
      n73 = Build Array(w200) -> (w193:refnum<class "Layer.lvclass">[])
      n74 = call-dynamic "SET_UserLayers.vi"("error in (no error)"=w195, "Layers"=w193, "Icon.lvclass in"=w201) -> ("error out"=w182:errorcluster, "Icon.lvclass out"=w183:refnum<class "Icon.lvclass">)  [unwired: 7 in]
      n75 = Bundle By Name(cluster=w184, "Class.Icon"=w183) -> (w181:T1)
      n76 = call "DeselectLayer.vi"("error in (no error)"=w182, "Data in"=w181) -> ("error out"=w177:errorcluster, "Data out"=w178:T1)  [unwired: 8 out]
      n77 = call "UpdateLayerView_ScrollbarChanged.vi"("error in"=w177, "Scrollbar Position"=0, "Data in"=w178) -> ("error out"=w175:errorcluster, "Data out"=w176:T1)  [unwired: 7 out]
    }
    frame "Merge Selected Layers" {
      n78 = Unbundle By Name(w236) -> ("Class.Icon"=w238:refnum<class "Icon.lvclass">, "Class.Layer"=w222:refnum<class "FakedArray.lvclass">)
      n79 = call-dynamic "GET_ActiveData.vi"("error in (no error)"=w219, "FakedArray in"=w222) -> ("error out"=w220:errorcluster, "Active Data []"=w218:i32[], "FakedArray out"=w221:refnum<class "FakedArray.lvclass">)  [unwired: 7 out]
      n80 = call-dynamic "GET_RowsCols.vi"("error in (no error)"=w220, "FakedArray.lvclass in"=w221) -> ("error out"=w230:errorcluster, "# Rows"=w229:i32)  [unwired: 8 out]
      n81 = call-dynamic "GET_UserLayers.vi"("error in (no error)"=w230, "Icon.lvclass in"=w238) -> ("error out"=w242:errorcluster, "All Layers"=w248:refnum<class "Layer.lvclass">[], "Icon.lvclass out"=w249:refnum<class "Icon.lvclass">)  [unwired: 7 out]
      n82 = call "Reset layer template selection.vi"("error in (no error)"=w242, "Data in"=w236) -> ("error out"=w241:errorcluster, "Data out"=w235:T1)  [unwired: 1 in, 7 out]
      n83 = Sort 1D Array(array=w218) -> (sorted array=w255:i32[])
      n84 = call "Separate Selected Layers.vi"("Active Indices"=w255, "All Layers"=w248) -> ("Layers out in Array"=w246:refnum<class "Layer.lvclass">[], "Layers out not in Array"=w247:refnum<class "Layer.lvclass">[])  [unwired: 8 out]
      n85 = Index Array(array=w255) -> (element=w227:i32)  [unwired: 1 in]
      n86 = call "Empty Picture"() -> ("empty picture"=w251:picture)
      n87 = for {
        shift-right: [w260] -> w253
        shift-left: w251 -> [w261]
        tunnel: w246 -> [w256] mode=indexing
        n88 = call-dynamic "GET_LayerData.vi"("Layer.lvclass in"=w256) -> ("Data"=w258:T11, "Origin"=w257:T5)  [unwired: 1 in, 8 out]
        n89 = Unbundle By Name(w258) -> ("Opacity"=w262:u8, "Visibility?"=w263:bool, "LayerIcon"=w259:picture)
        n90 = case shown="True" w263 {
          tunnel: w262 -> [_ w270]
          tunnel: w261 -> [w264 w269]
          tunnel: [w264 w268] -> w260
          tunnel: w259 -> [_ w267]
          tunnel: w257 -> [_ w266]
          frame False {
          }
          frame True {
            n91 = call "Draw Picture based on Origin.vi"("Origin"=w266, "LayerIcon in"=w267) -> ("LayerIcon out"=w265:picture)  [unwired: 1 in, 8 out]
            n92 = call "Apply Opacity.vi"("% (100)"=w270, "Bottom"=w269, "Top"=w265) -> ("new picture"=w268:picture)  [unwired: 8 out]
          }
        }
      }
      n93 = Bundle By Name(cluster=T11 {"LayerIcon"=bytes[0], "LayerName"="", "Opacity"=0, "Visibility?"=FALSE} ("Data"), "Opacity"=u8 100, "Visibility?"=TRUE, "LayerIcon"=w253, "LayerName"=w244) -> (w252:T11)
      n94 = call "Create default Layer.vi"() -> ("Layer.lvclass out"=w239:refnum<class "Layer.lvclass">)  [unwired: 1 in, 10 out]
      n95 = call-dynamic "SET_Layer_Data.vi"("error in (no error)"=w241, "Data"=w252, "Layer.lvclass in"=w239) -> ("error out"=w240:errorcluster, "Layer.lvclass out"=w250:refnum<class "Layer.lvclass">)  [unwired: 1 in, 6 out]
      n96 = Insert Into Array(array=w247, index=w227, new element=w250) -> (w245:refnum<class "Layer.lvclass">[])
      n97 = Subtract(x=w227, y=w229) -> (x-y=w228:i32)
      n98 = call-dynamic "SET_UserLayers.vi"("error in (no error)"=w240, "Layers"=w245, "Icon.lvclass in"=w249) -> ("error out"=w232:errorcluster, "Icon.lvclass out"=w237:refnum<class "Icon.lvclass">)  [unwired: 7 in]
      n99 = In Range and Coerce(upper limit=w227, x=w228, lower limit=0) -> (coerced(x)=w225:i32)  [unwired: 1 out]
      n100 = Bundle By Name(cluster=w235, "Class.Icon"=w237) -> (w234:T1)
      n101 = call "UpdateLayerView_ScrollbarChanged.vi"("error in"=w232, "Scrollbar Position"=w225, "Data in"=w234) -> ("error out"=w231:errorcluster, "Data out"=w233:T1)  [unwired: 7 out]
    }
    frame "Paste" {
      n102 = call "Empty Picture"() -> ("empty picture"=w276:picture)
      n103 = call "Import_Clipboard.vi"("error in (no error)"=w275, "Picture in"=w276) -> ("error out"=w274:errorcluster, "Valid?"=w273:bool, "Picture"=w272:picture)  [unwired: 1 in, 6 out]
      n104 = case shown="True" w273 {
        tunnel: [FALSE TRUE] -> w280
        tunnel: w279 -> [w282 w290]
        tunnel: [w283 w289] -> w278
        tunnel: [w282 w288] -> w277
        tunnel: w274 -> [w283 w287]
        tunnel: w272 -> [_ w286]
        tunnel: w271 -> [_ w284]
        frame False {
        }
        frame True {
          n105 = call "Create new layer_LayerName_Picture.vi"("error in"=w287, "Layer name"=w284, "Picture"=w286, "Data in"=w290) -> ("error out"=w289:errorcluster, "Data out"=w288:T1)  [unwired: 6 in]
        }
      }
    }
    frame "Import Glyph from File" {
      n106 = call "Load Glyph from File.vi"("error in (no error)"=w296) -> ("error out"=w295:errorcluster, "file name"=w292:string, "Pic Out"=w293:picture, "Canceled?"=w294:bool)  [unwired: 7 in]
      n107 = case shown="False" w294 {
        tunnel: w299 -> [w304 w307]
        tunnel: [w305 w308] -> w298
        tunnel: [w303 w307] -> w297
        tunnel: w295 -> [w306 w308]
        tunnel: w293 -> [w301 _]
        tunnel: w292 -> [w302 _]
        tunnel: [TRUE _] -> w291
        frame False {
          n108 = call "Create new layer_LayerName_Picture.vi"("error in"=w306, "Layer name"=w302, "Picture"=w301, "Data in"=w304) -> ("error out"=w305:errorcluster, "Data out"=w303:T1)  [unwired: 6 in]
        }
        frame True {
        }
      }
    }
    frame "Import Icon from Owning Library" {
      n109 = Unbundle By Name(w311) -> ("Class.Icon"=w319:refnum<class "Icon.lvclass">)
      n110 = call "Read Data from Caller.vi"("error in (no error)"=w321) -> ("error out"=w318:errorcluster, "Library Icon"=w316:picture)  [unwired: 5 in, 4 out]
      n111 = call-dynamic "GET_UserLayers.vi"("error in (no error)"=w318, "Icon.lvclass in"=w319) -> ("error out"=w313:errorcluster, "All Layers"=w317:refnum<class "Layer.lvclass">[], "Icon.lvclass out"=w315:refnum<class "Icon.lvclass">)  [unwired: 7 out]
      n112 = call "Create or Substitute NI_Layer layer.vi"("All Layers in"=w317, "new picture"=w316) -> ("All Layers out"=w314:refnum<class "Layer.lvclass">[])
      n113 = call-dynamic "SET_UserLayers.vi"("error in (no error)"=w313, "Layers"=w314, "Icon.lvclass in"=w315) -> ("error out"=w312:errorcluster, "Icon.lvclass out"=w310:refnum<class "Icon.lvclass">)  [unwired: 7 in]
      n114 = Bundle By Name(cluster=w311, "Class.Icon"=w310) -> (w309:T1)
    }
    frame "Redo", "Undo" {
      w345 = FALSE ("TM Set?")
      n115 = Unbundle By Name(w327) -> ("Class.Ants"=w326:refnum<class "Ants.lvclass">, "Ref.TextMarker"=w343:refnum<vi>)
      n116 = call "Const Temp Coordinate 2 points.vi"() -> ("Const Temp Coordinate"=w346:T5)  [unwired: 11 out]
      n117 = call "Const Temp Coordinate 4 points.vi"() -> ("Const Temp Coordinate"=w347:T21)  [unwired: 11 out]
      n118 = call "Empty Picture"() -> ("empty picture"=w344:picture)
      n119 = Bundle By Name(cluster=w327, "Support.Temp Icon"=w344, "Support.CTRL Pressed"=w345, "Support.Move Selection?"=w345, "Support.TM Set?"=w345, "Support.AntsRect"=w347, "Support.AntsRect Orig"=w347, "Support.Mouse Down Coords"=w346, "Support.Temp Coord"=w346) -> (w322:T1)
      n120 = Equal?(x=w340, y="Undo") -> (x = y?=w338:bool)
      n121 = property class="Str"(reference=w343, "Visible"=FALSE) -> ()  [unwired: 1 in, 2 out]
      n122 = Select(t=Undo_Redo_Action."Undo" ("Action"), s=w338, f=Undo_Redo_Action."Redo" ("Action")) -> (s? t:f=w335:T12)
      n123 = call "FireAntsEvent.vi"("error in (no error)"=w325, "Ants in"=w326) -> ("error out"=w341:errorcluster)  [unwired: 2 in, 7 out]
      n124 = call "FGV_Undo Redo.vi"("Action"=w335, "error in (no error)"=w341, "Data in"=w322) -> ("error out"=w334:errorcluster, 2:"Data out"=w328:string, 3:"Data out"=w324:T1)  [unwired: 1 in, 5 out]
      n125 = Unflatten From String(type=string[] [] ("appended array"), binary string=w328, error in (no error)=w334) -> (value=w332:string[], error out=w330:errorcluster)  [unwired: 2 in, 1 out]
      n126 = case shown="No Error" w330 {
        selector: w330 -> [w350 _]
        tunnel: w332 -> [w351 _]
        tunnel: [w352 _] -> w331
        tunnel: w324 -> [w349 w353]
        tunnel: [w348 w353] -> w323
        frame No Error {
          n127 = call "Replay Data from History.vi"("error in (no error)"=w350, 10:"Data in"=w351, 11:"Data in"=w349) -> ("error out"=w352:errorcluster, "Data out"=w348:T1)  [unwired: 5 in, 2 out]
        }
        frame Error {
          # "Do not\npropagate\nerror."
        }
      }
    }
    frame "Select All" {
      w376 = T22 {"Left"=0, "Top"=0, "Right"=32, "Bottom"=32} ("Rectangle")
      n128 = Unbundle By Name(w369) -> ("Class.Icon"=w361:refnum<class "Icon.lvclass">, "Class.Ants"=w370:refnum<class "Ants.lvclass">, "Ref.Tools"=w366:refnum<vi>, "Ref.Ants"=w375:refnum<vi>)
      n129 = property class="Pict"(reference=w375, error in=w373, "Visible"=TRUE) -> (error out=w364:errorcluster)  [unwired: 1 out]
      n130 = property class="RadioBtnsControl (strict)"(reference=w366, error in=w364, "Value"=T13."Select" ("Value (Signaling)")) -> (error out=w365:errorcluster)  [unwired: 1 out]
      n131 = call "Const Temp Coordinate 2 points.vi"() -> ("Const Temp Coordinate"=w372:T5)  [unwired: 11 out]
      n132 = call "FireAntsEvent.vi"("error in (no error)"=w365, "Rectangle (default: deselect)"=w376, "Ants in"=w370) -> ("error out"=w362:errorcluster)  [unwired: 1 in, 7 out]
      n133 = Bundle By Name(cluster=w369, "Support.CTRL Pressed"=FALSE, "Support.Tool (old value)"=u32 111, "Support.Mouse Move Coords"=w372, "Support.Mouse Down Coords"=w372, "Support.AntsRect"=w376, "Support.AntsRect Orig"=w376) -> (w356:T1)
      n134 = call-dynamic "GET_All User Layers.vi"("error in (no error)"=w362, "Icon.lvclass in"=w361) -> ("error out"=w357:errorcluster, "User Layer"=w360:refnum<class "Layer.lvclass">[])  [unwired: 7 in, 1 out]
      n135 = Array Size(array=w360) -> (size(s)=w359:i32)
      n136 = for {
        N: w359 -> [_]
        tunnel: [w377] -> w358 mode=indexing
        i -> [w377]
      }
      n137 = call "Set active Layer programmatically.vi"("error in"=w357, "Active Layer []"=w358, "Data in"=w356) -> ("error out"=w354:errorcluster, "Data out"=w355:T1)  [unwired: 7 in]
    }
    frame "Select Font", "Settings" {
      n138 = Equal?(x=w388, y="Select Font") -> (x = y?=w386:bool)
      n139 = Select(t="Text" ("y"), s=w386, f="") -> (s? t:f=w383:string)
      n140 = call "IconEditorSettings.vi"("error in (no error)"=w378, "Active Tag"=w383, "Data in"=w381) -> ("error out"=w380:errorcluster, "Data out"=w379:T1)  [unwired: 7 out]
    }
    frame "Select None" {
      n141 = call "Escape.vi"("error in"=w397, "Data in"=w396) -> ("error out"=w391:errorcluster, "Data out"=w392:T1)  [unwired: 2 in, 6 out]
      n142 = call "DeselectLayer.vi"("error in (no error)"=w391, "Data in"=w392) -> ("error out"=w394:errorcluster, "Data out"=w393:T1)  [unwired: 8 out]
      n143 = call "Reset layer template selection.vi"("error in (no error)"=w394, "Data in"=w393) -> ("error out"=w390:errorcluster, "Data out"=w389:T1)  [unwired: 1 in, 7 out]
    }
    frame "Show Layers Tab" {
      # "Changing the value of a tab control\nwhile FP updates are defered, does update\nthe value of the tab control (it even displays the\ncorrect content of the tab) but the tab\nselector stays on the old tab"
      n144 = call "Defer_FP_Updates.vi"("Defer Panel Updates"=FALSE, "error in (no error)"=w400, "lv_icon.vi in"=w399) -> ("error out"=w398:errorcluster)  [unwired: 8 out]
      n145 = Unbundle By Name(w405) -> ("Class.Settings"=w406:refnum<class "Settings.lvclass">)
      n146 = call-dynamic "GET_Show.vi"("error in (no error)"=w398, "Settings.lvclass in"=w406) -> ("error out"=w410:errorcluster, "Show Terminals?"=w412:bool, "Show LayerTab?"=w411:bool, "Settings.lvclass out"=w413:refnum<class "Settings.lvclass">)  [unwired: 6 out]
      n147 = Not(x=w411) -> (.not. x?=w407:bool)
      n148 = call "ShowLayersPalette.vi"("error in"=w410, "Show Layer Tab?"=w407, "Data in"=w405) -> ("error out"=w409:errorcluster)  [unwired: 8 out]
      n149 = call-dynamic "SET_Show.vi"("error in (no error)"=w409, "Show Terminals?"=w412, "Show Layer Tab?"=w407, "Settings.lvclass in"=w413) -> ("error out"=w402:errorcluster, "Settings.lvclass out"=w404:refnum<class "Settings.lvclass">)  [unwired: 6 out]
      n150 = Bundle By Name(cluster=w405, "Class.Settings"=w404) -> (w403:T1)
    }
    frame "Show Terminals" {
      n151 = Unbundle By Name(w419) -> ("Class.Settings"=w420:refnum<class "Settings.lvclass">)
      n152 = call-dynamic "GET_Show.vi"("error in (no error)"=w415, "Settings.lvclass in"=w420) -> ("error out"=w426:errorcluster, "Show Terminals?"=w423:bool, "Settings.lvclass out"=w428:refnum<class "Settings.lvclass">)  [unwired: 7 out]
      n153 = Not(x=w423) -> (.not. x?=w424:bool)
      n154 = call "ShowTerminals.vi"("Set Pic? (T)"=TRUE, "error in"=w426, "Tag enabled?"=TRUE, "Show Terminals?"=w424, "Data in"=w419) -> ("error out"=w425:errorcluster, "Data out"=w418:T1)  [unwired: 1 in, 4 out]
      n155 = call-dynamic "SET_Show.vi"("error in (no error)"=w425, "Show Terminals?"=w424, "Settings.lvclass in"=w428) -> ("error out"=w416:errorcluster, "Settings.lvclass out"=w417:refnum<class "Settings.lvclass">)  [unwired: 1 in, 6 out]
      n156 = Bundle By Name(cluster=w418, "Class.Settings"=w417) -> (w414:T1)
    }
    frame "Synchronize with Icon Library" {
      n157 = vi-ref "ni.com_iconlibrary.vi"() -> (w440:refnum<vi>)
      n158 = property class="VI"(reference=w440, error in=w438) -> (error out=w437:errorcluster, "Path"=w439:path)  [unwired: 1 out]
      n159 = Open VI Reference(vi path=w439, error in (no error)=w437) -> (vi reference=w441:refnum<vi>, error out=w442:errorcluster)  [unwired: 4 in]
      n160 = invoke class="VI" method="Run VI"(reference=w441, error in=w442, "Wait until done"=TRUE ("Wait Until Done"), "Auto Dispose Ref"=FALSE ("Auto Dispose Reference")) -> (reference out=w433:refnum<vi>, error out=w434:errorcluster)  [unwired: 1 in, 3 out]
      n161 = Close Reference(reference=w433, error in (no error)=w434) -> (error out=w431:errorcluster)
      n162 = Unbundle By Name(w431) -> ("code"=w432:i32)
      n163 = case shown="0, Default" w432 {
        tunnel: [w451 errorcluster {"status"=FALSE, "code"=0, "source"=""} ("error out")] -> w445
        tunnel: w443 -> [w450 _]
        tunnel: w431 -> [w449 _]
        tunnel: w430 -> [w448 w453]
        tunnel: [w448 w453] -> w429
        frame 0, Default {
          n164 = Unbundle By Name(w448) -> ("Ref.GlyphLoadAnimation"=w446:refnum<vi>, "Ref.refreshGlyphs"=w447:refnum<vi>)
          n165 = call "Launch Dynamically Load Graphics.vi"("User events"=w450, "Path"=Pathes."Glyphs", "error in (no error)"=w449, "button ref"=w447, "animatedDecoration ref"=w446) -> ("error out"=w451:errorcluster)  [unwired: 1 in, 5 out]
        }
        frame 1039 {
          # "VI was aborted"
        }
      }
    }
    frame "Template" {
      n166 = call "DrawIcon.vi"("Tools"=Tools."Ellipse", "error in (no error)"=w461, "Data in"=w466) -> ("error out"=w473:errorcluster, "Icon"=w472:picture, "Data out"=w457:T1)  [unwired: 2 in, 4 out]
      n167 = call "Read Data from Caller.vi"() -> ("Icon Editor Invoker Type"=w468:T23)  [unwired: 3 in, 8 out]
      n168 = call "Specify Path Enum.vi"("Icon Editor Invoker Type"=w468) -> ("Path"=w467:T9)  [unwired: 10 out]
      n169 = call "Get LV Glyph Path.vi"("Path"=w467, "error in (no error)"=w473) -> ("error out"=w465:errorcluster, "Requested Path"=w462:path)  [unwired: 1 in, 7 out]
      n170 = call "Get Image Data.vi"("Pic In"=w472) -> ("image data out"=w471:T15)  [unwired: 3 in, 7 out]
      n171 = call "Save Graphic.vi"("Loc string caption"=w458, "FP Title"=w463, "error in (no error)"=w465, "Start path in"=w462) -> ("error out"=w464:errorcluster, "Output"=w455:path)  [unwired: 6 out]
      n172 = Empty String/Path?(string/path=w455) -> (empty?=w459:bool)
      n173 = case shown="False" w459 {
        tunnel: w471 -> [w486 _]
        tunnel: w469 -> [w483 _]
        tunnel: w467 -> [w477 _]
        tunnel: w464 -> [w482 w490]
        tunnel: w455 -> [w476 _]
        tunnel: [w481 w490] -> w460
        tunnel: w457 -> [w480 w489]
        tunnel: [w480 w489] -> w456
        frame False {
          n174 = flat-sequence {
            tunnel: w476 -> [w488]
            tunnel: [w488] -> w475
            frame #0 {
              # "If the user pathologically deleted the specified folder while the dialog was up, this code will ensure that the owning folder exists when trying to save the .png file."
              n175 = Strip Path(path=w488) -> (stripped path=w487:path)  [unwired: 1 out]
              n176 = call <vilib>:"Create Directory Recursive.vi"("directory"=w487) -> ()  [unwired: 4 in, 3 out]
            }
          }
          n177 = Unbundle By Name(w480) -> ("Ref.TemplateLoadAnimation"=w479:refnum<vi>, "Ref.refreshTemplates"=w478:refnum<vi>)
          n178 = call <vilib>:"Write PNG File.vi"("error in (no error)"=w482, "image data"=w486, "path to PNG file"=w475) -> ("error out"=w485:errorcluster)  [unwired: 1 in, 7 out]
          n179 = call "Launch Dynamically Load Graphics.vi"("User events"=w483, "Template saved?"=TRUE, "Path"=w477, "error in (no error)"=w485, "button ref"=w478, "animatedDecoration ref"=w479) -> ("error out"=w481:errorcluster)  [unwired: 5 out]
        }
        frame True {
        }
      }
    }
    frame Default {
    }
  }
  n180 = call "ViewLayer.vi"("Add to Undo?"=w13, "error in (no error)"=w16, "Data in"=w14) -> ("error out"=w6:errorcluster, "Data out"=→"Data out":T1)  [unwired: 1 in, 6 out]
  n181 = call "Defer_FP_Updates.vi"("Defer Panel Updates"=FALSE, "error in (no error)"=w6, "lv_icon.vi in"=w4) -> ("error out"=→"error out":errorcluster)  [unwired: 8 out]
